vi "OP500Z8_Param_ConfZENplusOP100.vi"(8 "errin":errorcluster, 10 "Chaîne":string, 11 "pathin":path) -> (0 "errout":errorcluster, 3 "VISA OUT":T1)   [LabVIEW 2020]
uses:
  <vilib>/Utility/config.llb/Read Key (String).vi
  <vilib>/Utility/config.llb/NI_LVConfig.lvlib
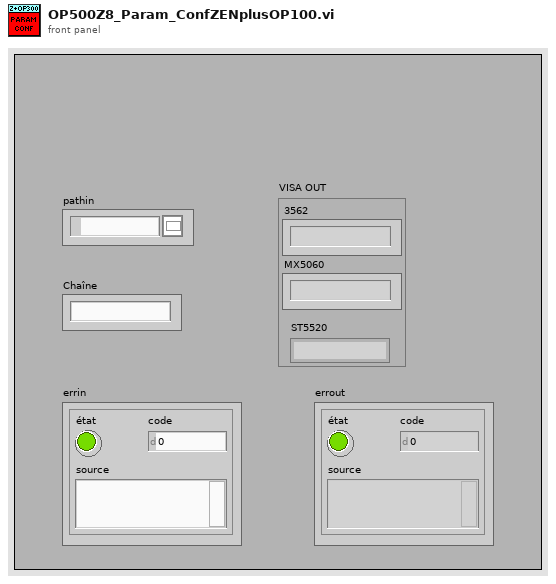
[diagram p1: front panel]
types:
  T1 = cluster{"3562":string, "MX5060":string, "ST5520":string}
  T2 = typedef "NI_LVConfig.lvlib/Config Data RefNum.ctl" = refnum<k1>
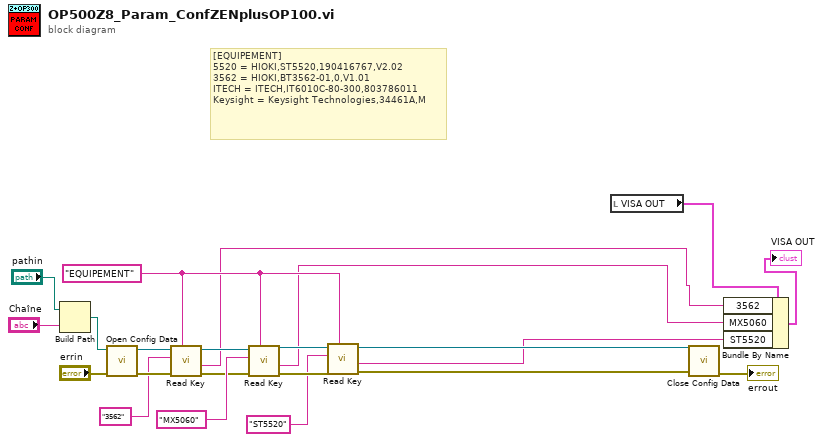
[diagram p0: block diagram]
diagram:
  w7 = "EQUIPEMENT" ("section")
  # "[EQUIPEMENT]\n5520 = HIOKI,ST5520,190416767,V2.02\n3562 = HIOKI,BT3562-01,0,V1.01\nITECH = ITECH,IT6010C-80-300,803786011\nKeysight = Keysight Technologies,34461A,M"
  n1 = Build Path(base path="pathin", name or relative path="Chaîne") -> (appended path=w19:path)
  n2 = call <vilib>:"Open Config Data.vi"("error in (no error)"="errin", "configuration file path"=w19) -> ("error out"=w21:errorcluster, "refnum"=w22:T2)  [unwired: 7 in, 1 out]
  n3 = call-poly <vilib>:"Read Key.vi"("section"=w7, "error in (no error)"=w21, "key"="3562", "refnum"=w22) -> ("error out"=w15:errorcluster, "value"=w4:string, "refnum out"=w18:T2)  [unwired: 4 in, 1 out]
  n4 = call-poly <vilib>:"Read Key.vi"("section"=w7, "error in (no error)"=w15, "key"="MX5060", "refnum"=w18) -> ("error out"=w11:errorcluster, "value"=w3:string, "refnum out"=w9:T2)  [unwired: 4 in, 1 out]
  n5 = call-poly <vilib>:"Read Key.vi"("section"=w7, "error in (no error)"=w11, "key"="ST5520", "refnum"=w9) -> ("error out"=w10:errorcluster, "value"=w2:string, "refnum out"=w8:T2)  [unwired: 4 in, 1 out]
  n6 = local read "VISA OUT"() -> (w5:T1)
  n7 = call <vilib>:"Close Config Data.vi"("error in (no error)"=w10, "refnum"=w8) -> ("error out"=→"errout":errorcluster)  [unwired: 8 in, 1 out]
  n8 = Bundle By Name(cluster=w5, "3562"=w4, "MX5060"=w3, "ST5520"=w2) -> (→"VISA OUT":T1)
